vi "GrapRoi.vi"() -> ()   [LabVIEW 2013]
panel:
  in  "ROI Ready":bool
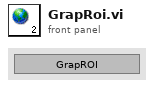
[diagram p1: front panel]
diagram:
